vi "mobile test.vi"() -> ()   [LabVIEW 2015]
uses:
  <vilib>/Utility/xml.llb/Write to XML File(string).vi
  <vilib>/Utility/file.llb/Write To Spreadsheet File (DBL).vi
panel:
  in  "HOW MANY TEST":i32
  in  "Name of File":string
  in  "FOLDER NAME":string
  out "String":string
  out "Numeric":dbl
  out "Waveform Chart":dbl(graph)
  in  "stop":bool
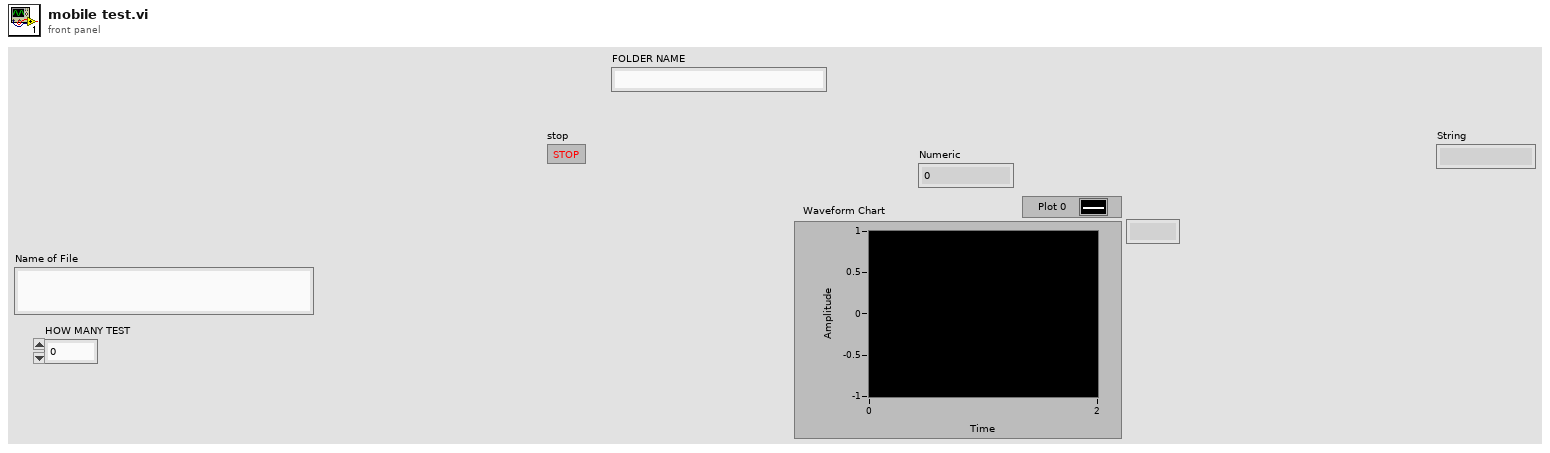
[diagram p1: front panel]
types:
  T1 = enum16{"open", "replace", "create", "open or create", "replace or create", "replace or create with confirmation"}
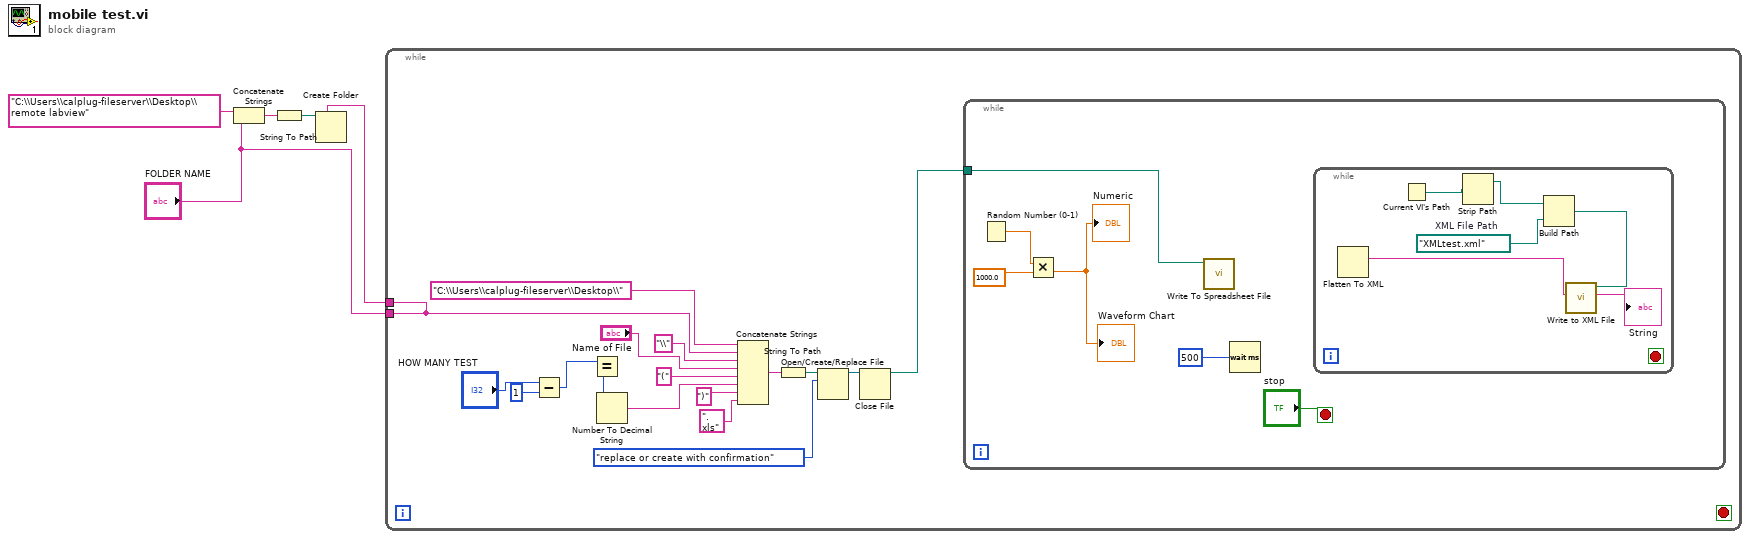
[diagram p0: block diagram]
diagram:
  n1 = Concatenate Strings("C:\\Users\\calplug-fileserver\\Desktop\\remote labview" ("string"), "FOLDER NAME") -> (w5:string)
  n2 = String To Path(string=w5) -> (path=w4:path)
  n3 = while {
    tunnel: [w7] -> w2
    tunnel: "FOLDER NAME" -> [w7]
    stop <- _ stop-if-true
    n4 = Subtract(x="HOW MANY TEST", y=1) -> (x-y=w8:i32)
    n5 = Number To Decimal String() -> (number=w11:i32, decimal integer string=w16:string)  [unwired: 1 in]
    n6 = Equal?(x=w8, y=w11) -> (x = y?=w12:bool)
    n7 = Concatenate Strings("C:\\Users\\calplug-fileserver\\Desktop\\" ("string"), w7, "\\" ("string"), "Name of File", "(" ("string"), w16, ")" ("string"), ".xls" ("string")) -> (w21:string)
    n8 = String To Path(string=w21) -> (path=w22:path)
    n9 = Open/Create/Replace File(file path (use dialog)=w22, operation (0:open)=T1."replace or create with confirmation") -> (refnum out=w20:refnum<file>)  [unwired: 4 in, 2 out]
    n10 = Close File(refnum=w20) -> (path=w6:path)  [unwired: 1 in, 1 out]
    n11 = while {
      tunnel: w6 -> [w25]
      stop <- "stop" stop-if-true
      n12 = Random Number (0-1)() -> (number: 0 to 1=w28:dbl)
      n13 = Multiply(x=w28, y=1000.0 ("number (0 to 1)")) -> (x*y=→"Waveform Chart" →"Numeric":dbl)
      n14 = call-poly <vilib>:"Write To Spreadsheet File.vi"("file path (dialog if empty)"=w25) -> ()  [unwired: 7 in, 1 out]
      n15 = Wait (ms)(milliseconds to wait=500) -> ()  [unwired: 1 out]
      n16 = while {
        stop <- _ stop-if-true
        w32 = path "XMLtest.xml"  # XML File Path
        n17 = Flatten To XML() -> (xml string=w30:string)  [unwired: 1 in]
        n18 = Current VI's Path() -> (path=w33:path)
        n19 = Strip Path(path=w33) -> (stripped path=w34:path)  [unwired: 1 out]
        n20 = Build Path(base path=w34, name or relative path=w32) -> (appended path=w35:path)
        n21 = call-poly <vilib>:"Write to XML File.vi"("XML Input"=w30, "XML File Path"=w35) -> ("XML String"=→"String":string)  [unwired: 7 in, 2 out]
      }
    }
  }
  n22 = Create Folder(prompt (Create Folder)=w2, path (use dialog)=w4) -> ()  [unwired: 1 in, 3 out]
